vi "ReadAPD.vi"() -> ()   [LabVIEW 2019]
uses:
  <vilib>/DAQmx/read.llb/DAQmx Read (Analog Wfm 1Chan NSamp).vi
  <vilib>/DAQmx/create/channels.llb/DAQmx Create Channel (AI-Voltage-Basic).vi
  <vilib>/DAQmx/miscellaneous.llb/DAQmx Fill In Error Info.vi
  <resource>/objmgr/daqmx.rc
panel:
  in  "Lockin Sensitivity":dbl=1000.0 format="%#_3p"
  out "APD Signal":waveform(dbl)(graph)
  in  "?":bool
  in  "Sampling Clock":dbl=1000.0 format="%#_3p"
  in  "Input Channel":tag="PXI1Slot8/ai0"
  # "(10 for default)"
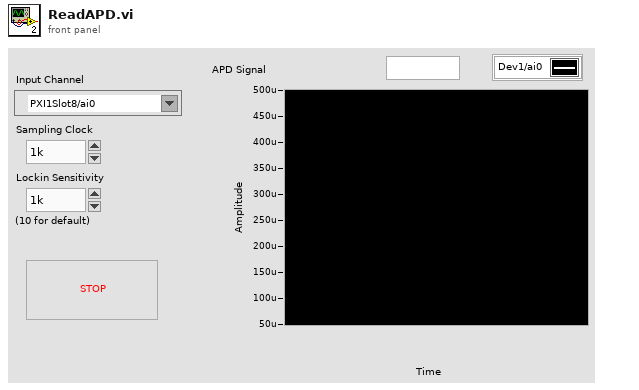
[diagram p1: front panel]
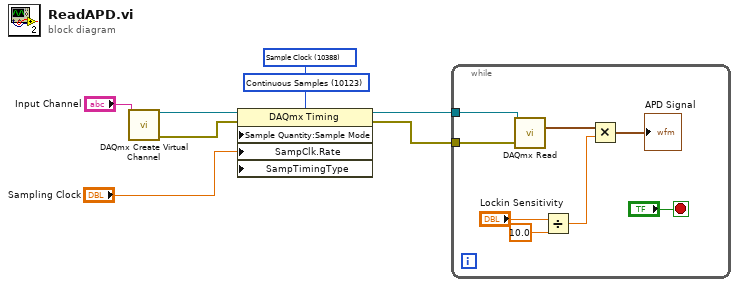
[diagram p0: block diagram]
diagram:
  w2 = 10388 items=["Sample Clock"=10388, "Burst Handshake"=12548, "Handshake"=10389, "Implicit"=10451, "On Demand"=10390, "Change Detection"=12504, "Pipelined Sample Clock"=14668] ("SampTimingType")
  w3 = 10123 items=["Finite Samples"=10178, "Continuous Samples"=10123, "Hardware Timed Single Point"=12522] ("SampQuant.SampMode")
  n1 = call-poly <vilib>:"DAQmx Create Virtual Channel.vi"("physical channels"="Input Channel") -> ("task out"=w7:refnum<k21>, "error out"=w5:errorcluster)  [unwired: 13 in]
  n2 = property class="DAQmx Timing"(reference=w7, error in=w5, "Sample Quantity:Sample Mode"=w3, "SampClk.Rate"="Sampling Clock", "SampTimingType"=w2) -> (reference out=w6:refnum<k21>, error out=w4:errorcluster)
  n3 = while {
    tunnel: w6 -> [w16]
    tunnel: w4 -> [w15]
    stop <- "?" stop-if-true
    n4 = call-poly <vilib>:"DAQmx Read.vi"("task/channels in"=w16, "error in"=w15) -> ("data"=w11:waveform(dbl))  [unwired: 11 in, 2 out]
    n5 = Divide(x="Lockin Sensitivity", y=10.0) -> (x/y=w10:dbl)
    n6 = Multiply(x=w11, y=w10) -> (x*y=→"APD Signal":waveform(dbl))
  }
